vi "SPC_get_fifo_usage.vi"(8 "Error In":errorcluster, 10 "Module No":i16 min=0 max=7 step=1, 11 "DLL Path":path) -> (0 "Error Out":errorcluster, 2 "Module No":i16 min=0 max=7 step=1, 3 "DLL Path":path, 4 "FIFO Usage Degree":sgl min=0 max=1 step=0.1 format="%.3f", 5 "FIFO usable":bool)   [LabVIEW 2017]
doc: "The procedure works only for SPC-13x/140/830/6x0/930/15x/160 modules in fifo mode.\nThe procedure sets \"usage_degree\" with the value in the range from 0 to 1, which tells how occupied is FIFO memory on the SPC module ‘mod_no’. \nFIFO memory usage is set to 0 at the start of FIFO measurement ( in SPC_start_measurement) and after reading data from FIFO ( SPC_read_fifo). \n\ninfo@becker-hickl.com"
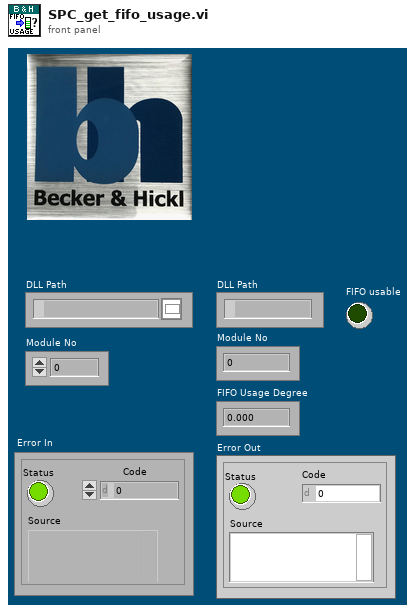
[diagram p1: front panel]
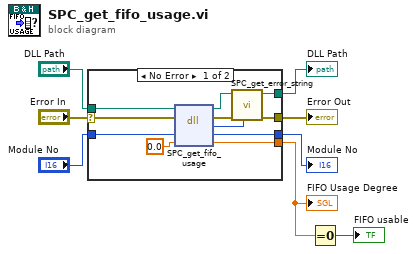
[diagram p0: block diagram]
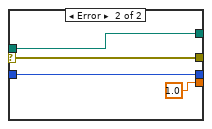
[diagram p2: hidden frame]
diagram:
  n1 = case shown="No Error" "Error In" {
    selector: "Error In" -> [w19 w23]
    tunnel: "DLL Path" -> [w18 w22]
    tunnel: [w13 w22] -> w6
    tunnel: [w16 w23] -> w5
    tunnel: [w12 sgl 1.0] -> w2
    tunnel: "Module No" -> [w11 w21]
    tunnel: [w10 w21] -> w3
    frame No Error {
      n2 = dll-call lib="D:/spcm/lib/lab_view/lv10.0/spcm32.dll" fn="SPC_get_fifo_usage"(path in=w18, error in=w19, "mod_no"=w11, "usage_degree"=sgl 0.0) -> (path out=w14:path, error out=w17:errorcluster, "return type"=w15:i16, "mod_no"=w10:i16, "usage_degree"=w12:sgl)  [unwired: 1 in]
      n3 = call "SPC_get_error_string.vi"("ErrorID"=w15, "Error In"=w17, "DLL Path"=w14) -> ("Error Out"=w16:errorcluster, "DLL Path"=w13:path)  [unwired: 6 in, 1 out]
    }
    frame Error {
    }
  }
  "DLL Path" <- w6
  "Error Out" <- w5
  "FIFO Usage Degree" <- w2
  "Module No" <- w3
  n4 = Equal To 0?(x=w2) -> (x = 0?=→"FIFO usable":bool)
